vi "Main.vi"(8 "error in (no error)":errorcluster, 11 "ModuleAdmin":refnum<class "ModuleAdmin.lvclass">) -> ()   [LabVIEW 2014, in "WfrmModule.lvlib"]
uses:
  WfrmModule.lvlib
  <userlib>/NIST/ModuleAdminLib/ModuleAdmin/ModuleAdmin.lvclass
  PublicAPI/Arguments/Requests/clStopArgument.ctl
  PublicAPI/Arguments/Requests/clLoadPlugin.ctl
  WfrmPlugins/EventPluginBaseClass/BaseWfrmPlugin.lvclass
  <userlib>/NIST/ModuleAdminLib/ModuleAdmin/ModuleAdmin.lvclass/ModuleAdmin.ctl
  WfrmPlugins/EventPluginBaseClass/TypeDefs/WfrmConfig.ctl
  PublicAPI/Arguments/Requests/clTimeParams.ctl
  WfrmPlugins/EventPluginBaseClass/BaseWfrmPlugin.lvclass/BaseWfrmPlugin.ctl
  PublicAPI/Arguments/Requests/dblEvtParams.ctl
  WfrmPlugins/EventPluginBaseClass/TypeDefs/clWfrmParams.ctl
  <vilib>/Utility/error.llb/DialogType.ctl
  <userlib>/NIST/ModuleAdminLib/ModuleAdmin/Accessors/Read ShowPanel_.vi
  WfrmPlugins/EventPluginBaseClass/Accessors/Write StartTime.vi
  WfrmPlugins/EventPluginBaseClass/Accessors/Write EndTime.vi
  WfrmPlugins/EventPluginBaseClass/Accessors/Write SettlingTime.vi
  WfrmPlugins/EventPluginBaseClass/Accessors/Read StartTime.vi
  WfrmPlugins/EventPluginBaseClass/Accessors/Read EndTime.vi
  WfrmPlugins/EventPluginBaseClass/Accessors/Read SettlingTime.vi
  WfrmPlugins/EventPluginBaseClass/Accessors/Write clWfrmParams.vi
  WfrmPlugins/EventPluginBaseClass/Accessors/Read clWfrmParams.vi
  <userlib>/NIST/ModuleAdminLib/ModuleAdmin/Accessors/Write ShowPanel_.vi
  <userlib>/NIST/ModuleAdminLib/ModuleAdmin/Accessors/Read CloneRegRef.vi
  <vilib>/Utility/error.llb/Error Cluster From Error Code.vi
  <vilib>/Analysis/1siggen.llb/Ramp Pattern by Delta.vi
  <vilib>/ErrorRing/Error Ring.xnode
  <userlib>/NIST/ModuleAdminLib/CloneRegistration/CloneRegistration.lvclass
  <vilib>/Analysis/NI_AALBase.lvlib
  <userlib>/NIST/ModuleAdminLib/ModuleAdmin.lvlib
  <userlib>/NIST/BaseClasses/Object_class/BaseObject.lvclass
panel:
  out "error out":errorcluster
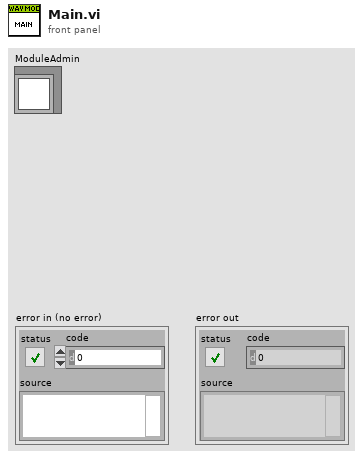
[diagram p1: front panel]
types:
  T1 = typedef "WfrmModule.lvlib/clRequestEvents.ctl" = cluster{"StopRequest":refnum<user-event>, "LoadPluginRequest":refnum<user-event>, "WriteEvtConfig":refnum<user-event>, "ReadEvtConfig":refnum<user-event>, "WriteTimeArray":refnum<user-event>, "ReadTimeArray":refnum<user-event>, "WriteEvtParams":refnum<user-event>, "ReadEvtParams":refnum<user-event>, "GetEvtReportArray":refnum<user-event>, "ReadPathToPlugin":refnum<user-event>, "GetEvtSignal":refnum<user-event>, "SendArbWfrm":refnum<user-event>, "ShowPanel":refnum<user-event>, "ReadWfrmParams":refnum<user-event>, "WriteWfrmParams":refnum<user-event>, "WriteStartEndTime":refnum<user-event>, "ConfigDlg":refnum<user-event>, "ReadStartEndSettlingTime":refnum<user-event>}
  T2 = typedef "WfrmModule.lvlib/clBroadcastEvents.ctl" = cluster{"DidInit":refnum<user-event>, "StatusUpdate":refnum<user-event>, "ErrorReport":refnum<user-event>, "DidStop":refnum<user-event>, "ReadEvtConfig":refnum<user-event>, "ReadTimeArray":refnum<user-event>, "ReadEvtParams":refnum<user-event>, "GetEvtReportArray":refnum<user-event>, "ReadPathToPlugin":refnum<user-event>, "GetEvtSignal":refnum<user-event>, "SendArbWfrm":refnum<user-event>, "WfrmParams":refnum<user-event>, "StartEndSettling":refnum<user-event>}
  T3 = typedef "WfrmModule.lvlib/clStopArgument.ctl" = cluster{"Exit via Stop Module Req?":bool, "Wait for Module to stop?":bool, "ModuleAdmin":refnum<class "ModuleAdmin.lvclass">}
  T4 = typedef "WfrmModule.lvlib/clLoadPlugin.ctl" = cluster{"PathToPlugin":path}
  T5 = enum32{"Invalid", "Standard", "Closed", "Hidden", "Minimized", "Maximized"}
  T6 = typedef "WfrmPlugins.lvlib/BaseWfrmPlugin.lvclass/WfrmConfig.ctl" = cluster{"T0(UTC)":dbl, "F0":dbl, "Fs":i32, "FSamp":u32}
  T7 = typedef "WfrmModule.lvlib/clTimeParams.ctl" = cluster{"dblTimeArray":dbl[], "StartTime":dbl, "EndTime":dbl, "SettlingTime":dbl}
  T8 = typedef "WfrmModule.lvlib/dblEvtParams.ctl" = dbl[][]
  T9 = typedef "WfrmPlugins.lvlib/BaseWfrmPlugin.lvclass/clWfrmParams.ctl" = cluster{"RowHdrs":string[], "ColHdrs":string[], "DefaultParams":string[][]}
  T10 = typedef "EventPlugins.lvlib/EventPluginBaseClass.lvclass/clEvtReportArray.ctl" = T11[]
  T11 = typedef "EventPlugins.lvlib/EventPluginBaseClass.lvclass/clEvtReport.ctl" = cluster{"Timestamp":dbl, "Synx":cdb[], "Freq":dbl, "ROCOF":dbl}
  T12 = typedef "EventModule.lvlib/dblEvtSignalArray.ctl" = dbl[][]
  T13 = typedef "DialogType.ctl" = u16
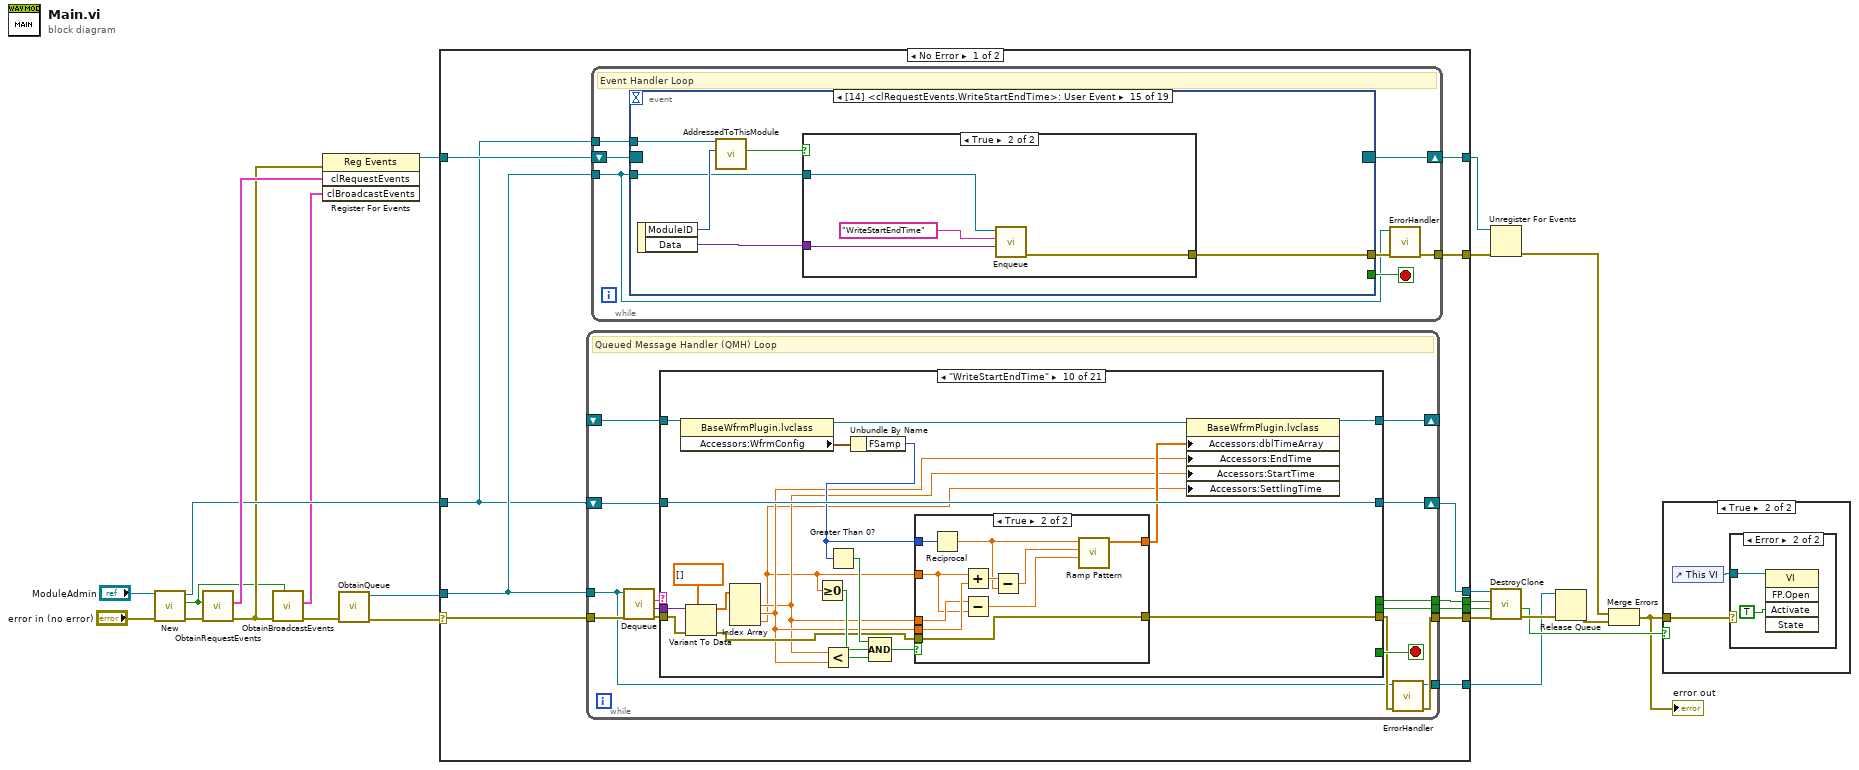
[diagram p0: block diagram]
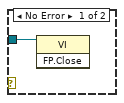
[diagram p3: hidden frame]
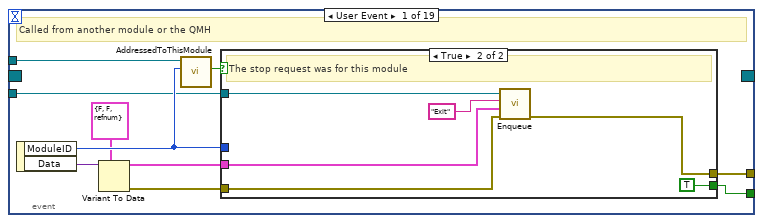
[diagram p4: hidden frame]
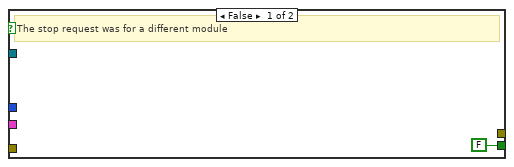
[diagram p5: hidden frame]
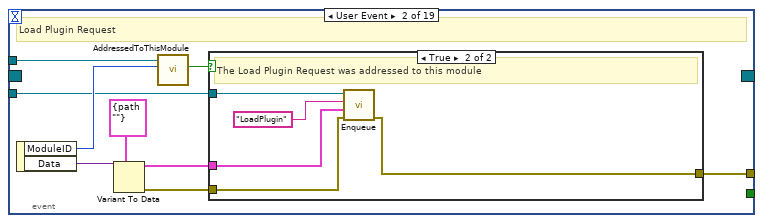
[diagram p6: hidden frame]
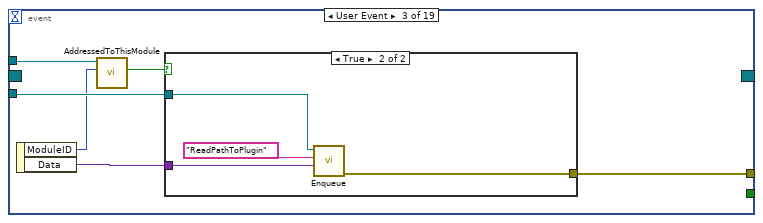
[diagram p8: hidden frame]
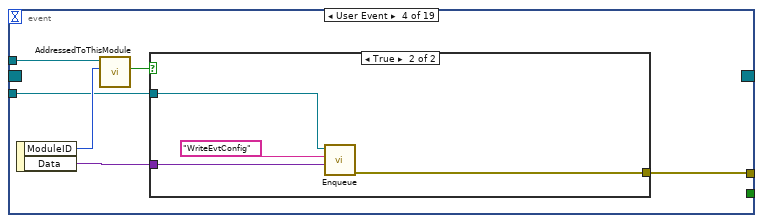
[diagram p10: hidden frame]
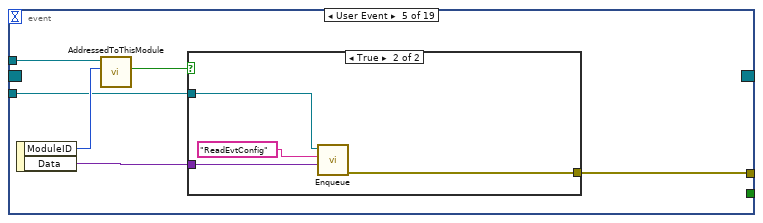
[diagram p12: hidden frame]
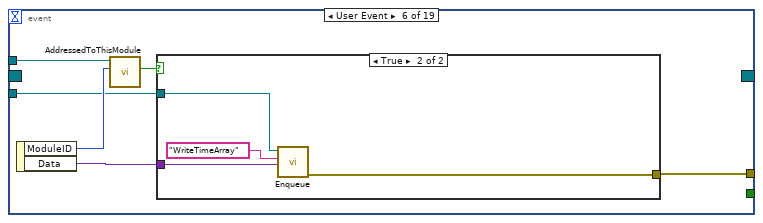
[diagram p14: hidden frame]
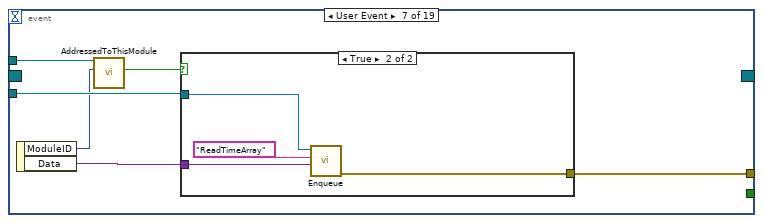
[diagram p16: hidden frame]
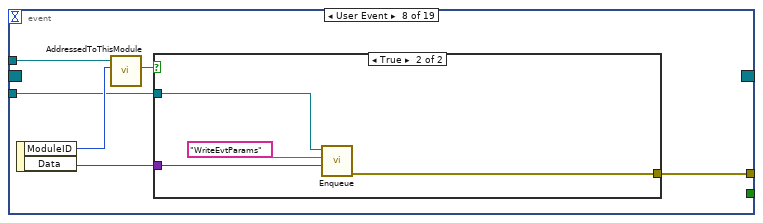
[diagram p18: hidden frame]
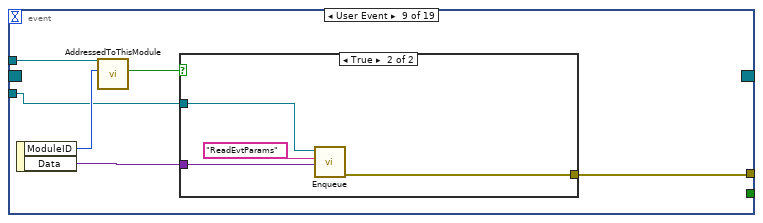
[diagram p20: hidden frame]
diagram:
  n1 = call <userlib>:"New.vi"("error in (no error)"="error in (no error)", "ModuleAdmin"="ModuleAdmin") -> ("error out"=w22:errorcluster, "First?"=w1:bool, "ModuleAdmin"=w18:refnum<class "ModuleAdmin.lvclass">)  [unwired: 7 in]
  n2 = call "ObtainRequestEvents.vi"("error in (no error)"=w22, "CreateNew (f)"=w1) -> ("error out"=w16:errorcluster, "clRequestEvents"=w21:T1)  [unwired: 8 in]
  n3 = call "ObtainBroadcastEvents.vi"("Init? (f)"=w1, "error in (no error)"=w16) -> ("error out"=w17:errorcluster, "clBroadcastEvents"=w15:T2)  [unwired: 8 in]
  n4 = register-events(error in=w16, w21, w15) -> (reference out=w14:refnum<event-registration>)  [unwired: 1 in, 1 out]
  n5 = call "ObtainQueue.vi"("error in (no error)"=w17) -> ("error out"=w20:errorcluster, "MessageQueue"=w19:refnum<queue>)  [unwired: 9 in]
  n6 = case shown="No Error" w20 {
    selector: w20 -> [w35 w635]
    tunnel: w19 -> [w33 w630]
    tunnel: w18 -> [w26 w632]
    tunnel: [w34 w633] -> w13
    tunnel: w14 -> [w32 w627]
    tunnel: [w31 w631] -> w11
    tunnel: [w30 _] -> w10
    tunnel: [w29 _] -> w9
    tunnel: [w28 _] -> w5
    tunnel: [w27 w630] -> w6
    tunnel: [w25 w627] -> w4
    frame No Error {
      n7 = while {
        tunnel: w33 -> [w252]
        tunnel: w35 -> [w260]
        tunnel: [w254] -> w34
        tunnel: [w256] -> w30
        tunnel: [w255] -> w29
        tunnel: [w251] -> w27
        shift-right: [w250] -> _
        shift-left: _ -> [w249]
        shift-right: [w248] -> w31
        shift-left: w26 -> [w247]
        stop <- w261 stop-if-true
        # "Queued Message Handler (QMH) Loop"
        n8 = call "Dequeue.vi"("error in (no error)"=w260, "MessageQueue"=w252) -> ("error out"=w259:errorcluster, "Message Data"=w257:variant, "Message"=w258:string)  [unwired: 6 in, 1 out]
        n9 = case shown="\"WriteStartEndTime\"" w258 {
          selector: w258 -> [w266 _ _ _ _ _ _ _ _ _ _ _ _ _ _ _ _ _ _ _ _]
          tunnel: [_ _ _ _ _ _ _ _ _ _ _ _ _ _ _ _ _ _ _ TRUE _] -> w261
          tunnel: w247 -> [w269 w298 w310 w359 w363 w375 w388 w399 w442 w467 w496 w508 w524 w535 w545 w562 w575 w588 w593 w601 w621]
          tunnel: [w265 w287 w311 w356 w365 w377 w386 w398 w441 w453 w498 w507 w523 w534 w544 w552 w565 w581 w591 w608 w612] -> w253
          tunnel: w259 -> [_ _ w321 w358 w367 w379 w383 w400 w443 w462 w499 w509 w525 w536 w546 w561 w574 w587 w599 w607 w620]
          tunnel: w257 -> [_ _ w325 _ _ w380 _ w401 _ w463 _ w510 w526 _ _ _ _ _ w600 w606 w619]
          tunnel: [_ _ _ _ _ _ _ _ _ _ _ _ _ _ _ _ _ _ _ w604 _] -> w256
          tunnel: [_ _ _ _ _ _ _ _ _ _ _ _ _ _ _ _ _ _ _ w603 _] -> w255
          tunnel: [w263 refnum<class "BaseWfrmPlugin.lvclass"> refnum ("EventPlugins.lvlib:EventPluginBaseClass.lvclass") w315 w357 w364 w376 w387 w397 w444 w465 w493 w505 w521 w533 w543 w558 w571 w584 w589 w602 w611] -> w250
          tunnel: w249 -> [w263 _ w316 w360 w366 w370 w389 w396 w445 w466 w503 w506 w522 w537 w547 w560 w573 w586 w589 w602 w611]
          tunnel: [w262 w282 w309 w354 w363 w368 w381 w392 w439 w467 w495 w504 w520 w532 w542 w550 w563 w576 w590 w601 w610] -> w248
          frame Default {
            n10 = property class="ModuleAdmin.lvclass"(reference=w269) -> (reference out=w262:refnum<class "ModuleAdmin.lvclass">, "Accessors:Module ID"=w268:i32, "Accessors:ModuleName"=w264:string)  [unwired: 1 in, 1 out]
            n11 = call <userlib>:"ModuleName.vi"("Name"=w264, "ModuleID"=w268) -> ("ModuleName"=w267:string)  [unwired: 9 in]
            n12 = xnode "Error Ring"("parameter 0"=w266, "parameter 1"=w267) -> ("error out"=w265:errorcluster)
          }
          frame "Initialize" {
            n13 = property class="ModuleAdmin.lvclass"(reference=w298) -> (reference out=w283:refnum<class "ModuleAdmin.lvclass">, error out=w295:errorcluster, "Accessors:Module ID"=w286:i32, "Accessors:ShowPanel_"=w280:bool, "Accessors:External Launch"=w279:bool, "Accessors:ModuleName"=w281:string)  [unwired: 1 in]
            n14 = Compound Arithmetic op=OR(w280, invert w279) -> (w278:bool)
            n15 = Select(t=T5."Standard" ("Front Panel Window:State"), s=w278, f=T5."Hidden" ("Front Panel Window:State")) -> (s? t:f=w291:T5)
            n16 = invoke class="VI" method="FP.Open"(error in=w295, "State"=w291) -> (error out=w294:errorcluster)  [unwired: 3 in, 4 out]
            n17 = call <userlib>:"ModuleName.vi"("Name"=w281, "ModuleID"=w286) -> ("ModuleName"=w290:string)  [unwired: 9 in]
            n18 = property class="VI"(error in=w294, "Front Panel.Title"=w290) -> (reference out=w297:refnum<vi>, error out=w296:errorcluster)  [unwired: 1 in]
            n19 = invoke class="VI" method="FP.Center"(reference=w297, error in=w296) -> (error out=w285:errorcluster)  [unwired: 1 in, 2 out]
            n20 = case shown="True" w279 {
              tunnel: [w299 w305] -> w288
              tunnel: [w300 w302] -> w282
              tunnel: w285 -> [w299 w304]
              tunnel: w283 -> [w300 w301]
              frame False {
              }
              frame True {
                n21 = call <userlib>:"WaitOnModuleSync.vi"("error in (no error)"=w304, "ModuleAdmin"=w301) -> ("error out"=w306:errorcluster, "ModuleAdmin"=w303:refnum<class "ModuleAdmin.lvclass">)  [unwired: 8 in]
                n22 = call <userlib>:"WaitOnEventSync.vi"("error in (no error)"=w306, "ModuleAdmin"=w303) -> ("error out"=w305:errorcluster, "ModuleAdmin"=w302:refnum<class "ModuleAdmin.lvclass">)  [unwired: 8 in]
              }
            }
            n23 = call "DidInit.vi"("Init?"=TRUE, "error in (no error)"=w288, "ModuleAdmin"=w282) -> ("error out"=w287:errorcluster)  [unwired: 8 in]
          }
          frame "LoadPlugin" {
            n24 = Variant To Data(error in=w321, type=T4 {"PathToPlugin"=path ""} ("clLoadPlugin"), Variant=w325) -> (data=w323:T4, error out=w322:errorcluster)
            n25 = Unbundle By Name(w323) -> ("PathToPlugin"=w308:path)
            n26 = call <userlib>:"GetPathToClass.vi"("error in (no error)"=w322, "configuration file path"=w308) -> ("error IO"=w320:errorcluster, "PathToClass"=w312:path)  [unwired: 8 in]
            n27 = Current VI's Path() -> (path=w313:path)
            n28 = Build Path(base path=w313, name or relative path=w312) -> (appended path=w314:path)
            n29 = call <vilib>:"Check if File or Folder Exists.vi"("error in (no error)"=w320, "path"=w314) -> ("error out"=w318:errorcluster, "file or folder exists?"=w319:bool, "dup path"=w317:path)  [unwired: 7 in]
            n30 = case shown="True" w319 {
              tunnel: w317 -> [w335 w342]
              tunnel: w318 -> [w339 w345]
              tunnel: [w334 w346] -> w311
              tunnel: w316 -> [_ w340]
              tunnel: w310 -> [w331 w341]
              tunnel: [w330 w341] -> w309
              tunnel: w308 -> [w327 _]
              tunnel: [w326 w340] -> w307
              frame True {
                n31 = call-dynamic "LoadClassFromFile.vi"("error in (no error)"=w339, "class path"=w335, "reference in"=refnum<class "BaseWfrmPlugin.lvclass"> refnum ("EventPlugins.lvlib:EventPluginBaseClass.lvclass")) -> ("error out"=w329:errorcluster, "reference out"=w328:refnum<class "BaseWfrmPlugin.lvclass">)  [unwired: 7 in]
                n32 = property class="ModuleAdmin.lvclass"(reference=w331) -> (reference out=w330:refnum<class "ModuleAdmin.lvclass">, "Accessors:Module ID"=w332:i32)  [unwired: 1 in, 1 out]
                n33 = call-dynamic "GetDefaultParams.vi"("error in (no error)"=w329, "ConfigFilePath"=w327, "BaseWfrmPlugin in"=w328) -> ("BaseWfrmPlugin out"=w326:refnum<class "BaseWfrmPlugin.lvclass">)  [unwired: 7 in, 1 out]
                n34 = Path To String(path=w335) -> (string=w337:string)
                n35 = Format Into String(format string="Plugin %s loaded", w337) -> (resulting string=w333:string)  [unwired: 2 in, 1 out]
                n36 = call "StatusUpdate.vi"("Status"=w333, "ModuleID"=w332) -> ("error out"=w334:errorcluster)  [unwired: 9 in]
              }
              frame False {
                n37 = Path To String(path=w342) -> (string=w343:string)
                n38 = xnode "Error Ring"("parameter 0"=w343) -> ("error out"=w344:errorcluster)
                n39 = Merge Errors(w344, w345) -> (w346:errorcluster)
              }
            }
            n40 = property class="BaseWfrmPlugin.lvclass"(reference=w307, "Accessors:EvtPluginINIFilePath"=w308) -> (reference out=w315:refnum<class "BaseWfrmPlugin.lvclass">)  [unwired: 1 in, 1 out]
          }
          frame "ReadPathToPlugin" {
            n41 = property class="BaseWfrmPlugin.lvclass"(reference=w360, error in=w358) -> (reference out=w357:refnum<class "BaseWfrmPlugin.lvclass">, error out=w361:errorcluster, "Accessors:EvtPluginINIFilePath"=w355:path)
            n42 = property class="ModuleAdmin.lvclass"(reference=w359) -> (reference out=w354:refnum<class "ModuleAdmin.lvclass">, "Accessors:Module ID"=w362:i32)  [unwired: 1 in, 1 out]
            n43 = call "ReadPathToPlugin.vi"("error in (no error)"=w361, "EvtPluginINIFilePath"=w355, "ModuleID"=w362) -> ("error out"=w356:errorcluster)  [unwired: 8 in]
          }
          frame "ConfigDlg" {
            n44 = call "ConfigureDlg.vi"("error in (no error)"=w367, "BaseWfrmPlugin in"=w366) -> ("error out"=w365:errorcluster, "BaseWfrmPlugin out"=w364:refnum<class "BaseWfrmPlugin.lvclass">)  [unwired: 8 in]
          }
          frame "WriteEvtConfig" {
            n45 = Variant To Data(error in=w379, type=T6 {"T0(UTC)"=0.0, "F0"=0.0, "Fs"=0, "FSamp"=0} ("clEvtConfig"), Variant=w380) -> (data=w371:T6, error out=w369:errorcluster)
            n46 = property class="BaseWfrmPlugin.lvclass"(reference=w370, error in=w369, "Accessors:WfrmConfig"=w371) -> (reference out=w376:refnum<class "BaseWfrmPlugin.lvclass">, error out=w372:errorcluster)
            n47 = property class="ModuleAdmin.lvclass"(reference=w375) -> (reference out=w368:refnum<class "ModuleAdmin.lvclass">, "Accessors:Module ID"=w374:i32)  [unwired: 1 in, 1 out]
            n48 = call "StatusUpdate.vi"("error in (no error)"=w372, "Status"="Event Configuration Received", "ModuleID"=w374) -> ("error out"=w377:errorcluster)  [unwired: 8 in]
          }
          frame "ReadEvtConfig" {
            n49 = property class="BaseWfrmPlugin.lvclass"(reference=w389, error in=w383) -> (reference out=w387:refnum<class "BaseWfrmPlugin.lvclass">, error out=w384:errorcluster, "Accessors:WfrmConfig"=w382:T6)
            n50 = property class="ModuleAdmin.lvclass"(reference=w388) -> (reference out=w381:refnum<class "ModuleAdmin.lvclass">, "Accessors:Module ID"=w385:i32)  [unwired: 1 in, 1 out]
            n51 = call "ReadEvtConfig.vi"("error in (no error)"=w384, "WfrmConfigReport"=w382, "ModuleID"=w385) -> ("error out"=w386:errorcluster)  [unwired: 8 in]
          }
          frame "WriteTimeArray" {
            n52 = Variant To Data(error in=w400, type=T7 {"dblTimeArray"=[], "StartTime"=0.0, "EndTime"=0.0, "SettlingTime"=7.0} ("clTimeParams"), Variant=w401) -> (data=w393:T7, error out=w395:errorcluster)
            n53 = Unbundle By Name(w393) -> ("dblTimeArray"=w390:dbl[])
            n54 = Array Size(array=w390) -> (size(s)=w394:i32)
            n55 = case shown="Default" w394 {
              tunnel: w399 -> [w409 w437]
              tunnel: [w412 w436] -> w398
              tunnel: [w419 w435] -> w397
              tunnel: w396 -> [w418 w432]
              tunnel: w395 -> [_ w431]
              tunnel: w393 -> [_ w430]
              tunnel: [w402 w429] -> w392
              frame 0, 1 {
                w415 = 0.0  # StartTime
                w416 = 1.0  # EndTime
                # "If the time array does not contain a valid time interval, set default time array and throw 5102 error."
                n56 = property class="BaseWfrmPlugin.lvclass"(reference=w418) -> (reference out=w417:refnum<class "BaseWfrmPlugin.lvclass">, error out=w414:errorcluster, "Accessors:WfrmConfig"=w405:T6)  [unwired: 1 in]
                n57 = property class="ModuleAdmin.lvclass"(reference=w409) -> (reference out=w402:refnum<class "ModuleAdmin.lvclass">, "Accessors:Module ID"=w408:i32)  [unwired: 1 in, 1 out]
                n58 = xnode "Error Ring"() -> ("error out"=w411:errorcluster)
                n59 = Unbundle By Name(w405) -> ("Fs"=w404:i32)
                n60 = Reciprocal(x=w404) -> (1/x=w406:dbl)
                n61 = call-poly <vilib>:"Ramp Pattern.vi"("start"=w415, "end"=w416, "delta"=w406) -> ("Ramp Pattern"=w403:dbl[])  [unwired: 6 in, 2 out]
                n62 = property class="BaseWfrmPlugin.lvclass"(reference=w417, error in=w414, "Accessors:dblTimeArray"=w403) -> (reference out=w419:refnum<class "BaseWfrmPlugin.lvclass">, error out=w410:errorcluster)
                n63 = call "StatusUpdate.vi"("error in (no error)"=w410, "Status"="Time Array invalid, setting 0 to 1 sec interval", "ModuleID"=w408) -> ("error out"=w413:errorcluster)  [unwired: 8 in]
                n64 = Merge Errors(w413, w411) -> (w412:errorcluster)
              }
              frame Default {
                n65 = Unbundle By Name(w430) -> ("dblTimeArray"=w428:dbl[], "StartTime"=w427:dbl, "EndTime"=w426:dbl, "SettlingTime"=w425:dbl)
                n66 = property class="BaseWfrmPlugin.lvclass"(reference=w432, error in=w431, "Accessors:dblTimeArray"=w428, "Accessors:StartTime"=w427, "Accessors:EndTime"=w426, "Accessors:SettlingTime"=w425) -> (reference out=w435:refnum<class "BaseWfrmPlugin.lvclass">, error out=w434:errorcluster)
                n67 = property class="ModuleAdmin.lvclass"(reference=w437) -> (reference out=w429:refnum<class "ModuleAdmin.lvclass">, "Accessors:Module ID"=w433:i32)  [unwired: 1 in, 1 out]
                n68 = call "StatusUpdate.vi"("error in (no error)"=w434, "Status"="Time Array Received", "ModuleID"=w433) -> ("error out"=w436:errorcluster)  [unwired: 8 in]
              }
            }
          }
          frame "ReadTimeArray" {
            n69 = property class="BaseWfrmPlugin.lvclass"(reference=w445, error in=w443) -> (reference out=w444:refnum<class "BaseWfrmPlugin.lvclass">, error out=w446:errorcluster, "Accessors:dblTimeArray"=w440:dbl[])
            n70 = property class="ModuleAdmin.lvclass"(reference=w442) -> (reference out=w439:refnum<class "ModuleAdmin.lvclass">, "Accessors:Module ID"=w447:i32)  [unwired: 1 in, 1 out]
            n71 = call "ReadTimeArray.vi"("error in (no error)"=w446, "dblTime Array"=w440, "ModuleID"=w447) -> ("error out"=w441:errorcluster)  [unwired: 8 in]
          }
          frame "WriteStartEndTime" {
            n72 = property class="BaseWfrmPlugin.lvclass"(reference=w466) -> (reference out=w464:refnum<class "BaseWfrmPlugin.lvclass">, "Accessors:WfrmConfig"=w459:T6)  [unwired: 1 in, 1 out]
            n73 = Variant To Data(error in=w462, type=dbl[] [], Variant=w463) -> (data=w460:dbl[], error out=w451:errorcluster)
            n74 = Index Array(array=w460) -> (element #1=w449:dbl, element #2=w450:dbl, element #3=w448:dbl)  [unwired: 3 in]
            n75 = Greater Or Equal To 0?(x=w448) -> (x >= 0?=w457:bool)
            n76 = Less?(x=w449, y=w450) -> (x < y?=w458:bool)
            n77 = Unbundle By Name(w459) -> ("FSamp"=w454:u32)
            n78 = Greater Than 0?(x=w454) -> (x > 0?=w456:bool)
            n79 = Compound Arithmetic op=AND(w456, w457, w458) -> (w455:bool)
            n80 = case shown="True" w455 {
              tunnel: w454 -> [w470 w492]
              tunnel: w448 -> [w469 w487]
              tunnel: w449 -> [w472 w488]
              tunnel: w450 -> [w471 w491]
              tunnel: [w468 w483] -> w453
              tunnel: [_ w484] -> w452
              tunnel: w451 -> [_ w483]
              frame False {
                n81 = xnode "Error Ring"("parameter 0"=w472, "parameter 1"=w471, "parameter 2"=w470, "parameter 3"=w469) -> ("error out"=w468:errorcluster)
              }
              frame True {
                n82 = Reciprocal(x=w492) -> (1/x=w489:dbl)
                n83 = Add(x=w487, y=w491) -> (x+y=w490:dbl)
                n84 = Subtract(x=w488, y=w487) -> (x-y=w485:dbl)
                n85 = Subtract(x=w490, y=w489) -> (x-y=w486:dbl)
                n86 = call-poly <vilib>:"Ramp Pattern.vi"("start"=w485, "end"=w486, "delta"=w489) -> ("Ramp Pattern"=w484:dbl[])  [unwired: 6 in, 2 out]
              }
            }
            n87 = property class="BaseWfrmPlugin.lvclass"(reference=w464, "Accessors:dblTimeArray"=w452, "Accessors:EndTime"=w450, "Accessors:StartTime"=w449, "Accessors:SettlingTime"=w448) -> (reference out=w465:refnum<class "BaseWfrmPlugin.lvclass">)  [unwired: 1 in, 1 out]
          }
          frame "ReadStartEndTime" {
            n88 = property class="BaseWfrmPlugin.lvclass"(reference=w503) -> (reference out=w493:refnum<class "BaseWfrmPlugin.lvclass">, "Accessors:StartTime"=w500:dbl, "Accessors:EndTime"=w501:dbl, "Accessors:SettlingTime"=w502:dbl)  [unwired: 1 in, 1 out]
            n89 = property class="ModuleAdmin.lvclass"(reference=w496) -> (reference out=w495:refnum<class "ModuleAdmin.lvclass">, "Accessors:Module ID"=w494:i32)  [unwired: 1 in, 1 out]
            n90 = Build Array(w500, w501, w502) -> (w497:dbl[])
            n91 = call "ReadStartEndSettling.vi"("error in (no error)"=w499, "StartEndSettling"=w497, "ModuleID"=w494) -> ("error out"=w498:errorcluster)  [unwired: 8 in]
          }
          frame "WriteEvtParams" {
            w511 = T8 []  # SignalParams
            # "Can't change \"SignalParams\" to icon."
            n92 = Variant To Data(error in=w509, type=w511, Variant=w510) -> (data=w512:T8, error out=w516:errorcluster)
            n93 = property class="BaseWfrmPlugin.lvclass"(reference=w506, error in=w516, "Accessors:dblEvtParams"=w512) -> (reference out=w505:refnum<class "BaseWfrmPlugin.lvclass">, error out=w513:errorcluster)
            n94 = property class="ModuleAdmin.lvclass"(reference=w508) -> (reference out=w504:refnum<class "ModuleAdmin.lvclass">, "Accessors:Module ID"=w515:i32)  [unwired: 1 in, 1 out]
            n95 = call "StatusUpdate.vi"("error in (no error)"=w513, "Status"="Event Parameters Received", "ModuleID"=w515) -> ("error out"=w507:errorcluster)  [unwired: 8 in]
          }
          frame "WriteWfrmParams" {
            w527 = T9 {"RowHdrs"=[], "ColHdrs"=[], "DefaultParams"=[]}  # SignalParams
            n96 = Variant To Data(error in=w525, type=w527, Variant=w526) -> (data=w518:T9, error out=w531:errorcluster)
            n97 = Unbundle By Name(w518) -> ("DefaultParams"=w517:string[][])
            n98 = call "Tbl2Array.vi"("strTable"=w517) -> ("dblArray"=w519:dbl[][])  [unwired: 10 in]
            n99 = property class="BaseWfrmPlugin.lvclass"(reference=w522, error in=w531, "Accessors:clWfrmParams"=w518, "Accessors:dblEvtParams"=w519) -> (reference out=w521:refnum<class "BaseWfrmPlugin.lvclass">, error out=w528:errorcluster)
            n100 = property class="ModuleAdmin.lvclass"(reference=w524) -> (reference out=w520:refnum<class "ModuleAdmin.lvclass">, "Accessors:Module ID"=w530:i32)  [unwired: 1 in, 1 out]
            n101 = call "StatusUpdate.vi"("error in (no error)"=w528, "Status"="Waveform Parameters Received", "ModuleID"=w530) -> ("error out"=w523:errorcluster)  [unwired: 8 in]
          }
          frame "ReadEvtParams" {
            n102 = property class="BaseWfrmPlugin.lvclass"(reference=w537, error in=w536) -> (reference out=w533:refnum<class "BaseWfrmPlugin.lvclass">, error out=w539:errorcluster, "Accessors:dblEvtParams"=w538:dbl[][])
            n103 = property class="ModuleAdmin.lvclass"(reference=w535) -> (reference out=w532:refnum<class "ModuleAdmin.lvclass">, "Accessors:Module ID"=w540:i32)  [unwired: 1 in, 1 out]
            n104 = call "ReadEvtParams.vi"("error in (no error)"=w539, "SignalParams"=w538, "ModuleID"=w540) -> ("error out"=w534:errorcluster)  [unwired: 8 in]
          }
          frame "ReadWfrmParams" {
            n105 = property class="BaseWfrmPlugin.lvclass"(reference=w547, error in=w546) -> (reference out=w543:refnum<class "BaseWfrmPlugin.lvclass">, error out=w548:errorcluster, "Accessors:clWfrmParams"=w541:T9)
            n106 = property class="ModuleAdmin.lvclass"(reference=w545) -> (reference out=w542:refnum<class "ModuleAdmin.lvclass">, "Accessors:Module ID"=w549:i32)  [unwired: 1 in, 1 out]
            n107 = call "WfrmParams.vi"("error in (no error)"=w548, "WfrmParams"=w541, "ModuleID"=w549) -> ("error out"=w544:errorcluster)  [unwired: 8 in]
          }
          frame "GetReportArray" {
            n108 = call-dynamic "GetEvtReports.vi"("error in (no error)"=w561, "EventPluginBaseClass in"=w560) -> ("error out"=w557:errorcluster, "EventPluginBaseClass out"=w559:refnum<class "BaseWfrmPlugin.lvclass">)  [unwired: 8 in]
            n109 = property class="ModuleAdmin.lvclass"(reference=w562) -> (reference out=w550:refnum<class "ModuleAdmin.lvclass">, "Accessors:Module ID"=w551:i32)  [unwired: 1 in, 1 out]
            n110 = property class="BaseWfrmPlugin.lvclass"(reference=w559, error in=w557) -> (reference out=w558:refnum<class "BaseWfrmPlugin.lvclass">, error out=w556:errorcluster, "Accessors:clEvtReportArray"=w555:T10)
            n111 = call "GetEvtReports.vi"("error in (no error)"=w556, "clReportArray"=w555, "ModuleID"=w551) -> ("error out"=w553:errorcluster)  [unwired: 8 in]
            n112 = call "StatusUpdate.vi"("error in (no error)"=w553, "Status"="Event Reports Transmitted", "ModuleID"=w551) -> ("error out"=w552:errorcluster)  [unwired: 8 in]
          }
          frame "GetEvtSignal" {
            n113 = call-dynamic "GetEvtSignal.vi"("error in (no error)"=w574, "EventPluginBaseClass in"=w573) -> ("error out"=w570:errorcluster, "EventPluginBaseClass out"=w572:refnum<class "BaseWfrmPlugin.lvclass">)  [unwired: 8 in]
            n114 = property class="ModuleAdmin.lvclass"(reference=w575) -> (reference out=w563:refnum<class "ModuleAdmin.lvclass">, "Accessors:Module ID"=w564:i32)  [unwired: 1 in, 1 out]
            n115 = property class="BaseWfrmPlugin.lvclass"(reference=w572, error in=w570) -> (reference out=w571:refnum<class "BaseWfrmPlugin.lvclass">, error out=w569:errorcluster, "Accessors:dblEventSignalArray"=w568:T12)
            n116 = call "GetEvtSignal.vi"("error in (no error)"=w569, "clReportArray"=w568, "ModuleID"=w564) -> ("error out"=w566:errorcluster)  [unwired: 8 in]
            n117 = call "StatusUpdate.vi"("error in (no error)"=w566, "Status"="Event Signal Transmitted", "ModuleID"=w564) -> ("error out"=w565:errorcluster)  [unwired: 8 in]
          }
          frame "SendArbWfrm" {
            n118 = call-dynamic "GetEvtSignal.vi"("error in (no error)"=w587, "EventPluginBaseClass in"=w586) -> ("error out"=w583:errorcluster, "EventPluginBaseClass out"=w585:refnum<class "BaseWfrmPlugin.lvclass">)  [unwired: 8 in]
            n119 = property class="ModuleAdmin.lvclass"(reference=w588) -> (reference out=w576:refnum<class "ModuleAdmin.lvclass">, "Accessors:Module ID"=w580:i32)  [unwired: 1 in, 1 out]
            n120 = property class="BaseWfrmPlugin.lvclass"(reference=w585, error in=w583) -> (reference out=w584:refnum<class "BaseWfrmPlugin.lvclass">, error out=w578:errorcluster, "Accessors:dblEventSignalArray"=w579:T12)
            n121 = call "SendEvtSignal.vi"("error in (no error)"=w578, "clReportArray"=w579, "ModuleID"=w580) -> ("error out"=w577:errorcluster)  [unwired: 8 in]
            n122 = call "StatusUpdate.vi"("error in (no error)"=w577, "Status"="Event Signal Transmitted", "ModuleID"=w580) -> ("error out"=w581:errorcluster)  [unwired: 8 in]
          }
          frame "ShowPanel" {
            n123 = Variant To Data(error in=w599, type=TRUE, Variant=w600) -> (data=w592:bool, error out=w594:errorcluster)
            n124 = Select(t=T5."Standard" ("Front Panel Window:State"), s=w592, f=T5."Hidden" ("Front Panel Window:State")) -> (s? t:f=w595:T5)
            n125 = property class="VI"(error in=w594, "FP.State"=w595) -> (error out=w591:errorcluster)  [unwired: 1 in, 1 out]
            n126 = property class="ModuleAdmin.lvclass"(reference=w593, "Accessors:ShowPanel_"=w592) -> (reference out=w590:refnum<class "ModuleAdmin.lvclass">)  [unwired: 1 in, 1 out]
          }
          frame "Exit" {
            n127 = control-ref of="This VI"() -> (w605:refnum<vi>)
            n128 = call "HandleExit.vi"("error in (no error)"=w607, "VI Refnum"=w605, "StopArgument"=w606, "ModuleAdmin"=w601) -> ("error out"=w608:errorcluster, "Exit via Stop Module Req?"=w603:bool, "WaitForStop?"=w604:bool)  [unwired: 5 in]
          }
          frame "Error" {
            n129 = property class="ModuleAdmin.lvclass"(reference=w621) -> (reference out=w610:refnum<class "ModuleAdmin.lvclass">, "Accessors:External Launch"=w615:bool, "Accessors:Module ID"=w613:i32)  [unwired: 1 in, 1 out]
            n130 = Variant To Data(error in=w620, type=errorcluster {"status"=FALSE, "code"=0, "source"=""} ("error constant"), Variant=w619) -> (data=w614:errorcluster, error out=w617:errorcluster)
            n131 = call "ReportError.vi"("error in (no error)"=w617, "ErrorReported"=w614, "ModuleID"=w613) -> ("error out"=w616:errorcluster)  [unwired: 8 in]
            n132 = case shown="True" w615 {
              tunnel: w616 -> [w625 w626]
              tunnel: w614 -> [w624 _]
              tunnel: [w623 w626] -> w612
              tunnel: w610 -> [w622 _]
              frame False {
                # "Todo:  Add an event to ask the user\nIf the module should stop or continue"
                # "Stand alone: now, force an exit"
                n133 = call <vilib>:"Simple Error Handler.vi"("error in (no error)"=w624) -> ()  [unwired: 4 in, 5 out]
                n134 = call "StopRequest.vi"("error in (no error)"=w625, "ModuleAdmin"=w622) -> ("error out"=w623:errorcluster)  [unwired: 8 in, 1 out]
              }
              frame True {
                # "Externally launched modules only broadcast the error msg"
              }
            }
          }
        }
        n135 = call "ErrorHandler.vi"("error in (no error)"=w253, "MessageQueue"=w252) -> ("error out"=w254:errorcluster, "MessageQueue"=w251:refnum<queue>)  [unwired: 8 in]
      }
      n136 = while {
        tunnel: w33 -> [w36]
        shift-right: [w40] -> w25
        shift-left: w32 -> [w41]
        tunnel: w26 -> [w39]
        tunnel: [w37] -> w28
        stop <- w42 stop-if-true
        # "Event Handler Loop"
        n137 = event shown="[14] <clRequestEvents.WriteStartEndTime>: User Event" {
          selector: w41 -> [_ _ _ _ _ _ _ _ _ _ _ _ _ _ _ _ _ _ _]
          dyn-events: [_ _ _ _ _ _ _ _ _ _ _ _ _ _ _ _ _ _ _] -> w40
          timeout: _ -> [_ _ _ _ _ _ _ _ _ _ _ _ _ _ _ _ _ _ _]
          tunnel: w36 -> [w49 w63 w77 w85 w95 w104 w117 w125 w135 w145 w155 w166 w176 w186 w196 w206 w216 w226 w246]
          tunnel: [w48 _ _ _ _ _ _ _ _ _ _ _ _ _ _ _ _ _ TRUE] -> w42
          tunnel: w39 -> [w52 w60 w78 w88 w99 w107 w118 w126 w137 w147 w157 w168 w178 w188 w198 w208 w218 w229 w240]
          tunnel: [w47 w62 w74 w84 w94 w108 w114 w124 w134 w144 w154 w164 w174 w184 w194 w204 w214 w224 w244] -> w38
          event User Event {
            # "Called from another module or the QMH"
            n138 = event-data() -> ("ModuleID"=w50:i32, "Data"=w46:variant)  [unwired: 1 in]
            n139 = Variant To Data(type=T3 {"Exit via Stop Module Req?"=FALSE, "Wait for Module to stop?"=FALSE, "ModuleAdmin"=refnum} ("Stop Argument"), Variant=w46) -> (data=w44:T3, error out=w43:errorcluster)  [unwired: 1 in]
            n140 = call <userlib>:"AddressedToThisModule.vi"("ModuleID"=w50, "ModuleAdmin"=w52) -> ("AddressedToThisInstance?"=w51:bool)  [unwired: 8 in, 1 out]
            n141 = case shown="True" w51 {
              tunnel: w50 -> [_ _]
              tunnel: w49 -> [_ w59]
              tunnel: [FALSE TRUE] -> w48
              tunnel: [_ w57] -> w47
              tunnel: w44 -> [_ w55]
              tunnel: w43 -> [_ w54]
              frame False {
                # "The stop request was for a different module"
              }
              frame True {
                # "The stop request was for this module"
                n142 = call "Enqueue.vi"("error in (no error)"=w54, "Message Data"=w55, "Message"="Exit", "MessageQueue"=w59) -> ("error out"=w57:errorcluster)  [unwired: 6 in, 1 out]
              }
            }
          }
          event User Event {
            # "Load Plugin Request"
            n143 = event-data() -> ("ModuleID"=w64:i32, "Data"=w68:variant)  [unwired: 1 in]
            n144 = Variant To Data(type=T4 {"PathToPlugin"=path ""} ("clLoadPlugin"), Variant=w68) -> (data=w65:T4, error out=w61:errorcluster)  [unwired: 1 in]
            n145 = call <userlib>:"AddressedToThisModule.vi"("ModuleID"=w64, "ModuleAdmin"=w60) -> ("AddressedToThisInstance?"=w66:bool)  [unwired: 8 in, 1 out]
            n146 = case shown="True" w66 {
              tunnel: w65 -> [_ w73]
              tunnel: w63 -> [_ w72]
              tunnel: [_ w70] -> w62
              tunnel: w61 -> [_ w69]
              frame False {
                # "Not addressed to this module"
              }
              frame True {
                # "The Load Plugin Request was addressed to this module"
                n147 = call "Enqueue.vi"("error in (no error)"=w69, "Message Data"=w73, "Message"="LoadPlugin", "MessageQueue"=w72) -> ("error out"=w70:errorcluster)  [unwired: 6 in, 1 out]
              }
            }
          }
          event User Event {
            n148 = event-data() -> ("ModuleID"=w76:i32, "Data"=w75:variant)  [unwired: 1 in]
            n149 = call <userlib>:"AddressedToThisModule.vi"("ModuleID"=w76, "ModuleAdmin"=w78) -> ("AddressedToThisInstance?"=w79:bool)  [unwired: 8 in, 1 out]
            n150 = case shown="True" w79 {
              tunnel: w75 -> [_ w83]
              tunnel: w77 -> [_ w82]
              tunnel: [_ w80] -> w74
              frame False {
              }
              frame True {
                n151 = call "Enqueue.vi"("Message Data"=w83, "Message"="ReadPathToPlugin", "MessageQueue"=w82) -> ("error out"=w80:errorcluster)  [unwired: 7 in, 1 out]
              }
            }
          }
          event User Event {
            n152 = event-data() -> ("ModuleID"=w89:i32, "Data"=w86:variant)  [unwired: 1 in]
            n153 = call <userlib>:"AddressedToThisModule.vi"("ModuleID"=w89, "ModuleAdmin"=w88) -> ("AddressedToThisInstance?"=w87:bool)  [unwired: 8 in, 1 out]
            n154 = case shown="True" w87 {
              tunnel: w86 -> [_ w93]
              tunnel: w85 -> [_ w91]
              tunnel: [_ w90] -> w84
              frame False {
              }
              frame True {
                n155 = call "Enqueue.vi"("Message Data"=w93, "Message"="WriteEvtConfig", "MessageQueue"=w91) -> ("error out"=w90:errorcluster)  [unwired: 7 in, 1 out]
              }
            }
          }
          event User Event {
            n156 = event-data() -> ("ModuleID"=w98:i32, "Data"=w97:variant)  [unwired: 1 in]
            n157 = call <userlib>:"AddressedToThisModule.vi"("ModuleID"=w98, "ModuleAdmin"=w99) -> ("AddressedToThisInstance?"=w96:bool)  [unwired: 8 in, 1 out]
            n158 = case shown="True" w96 {
              tunnel: w97 -> [_ w103]
              tunnel: w95 -> [_ w102]
              tunnel: [_ w100] -> w94
              frame False {
              }
              frame True {
                n159 = call "Enqueue.vi"("Message Data"=w103, "Message"="ReadEvtConfig", "MessageQueue"=w102) -> ("error out"=w100:errorcluster)  [unwired: 7 in, 1 out]
              }
            }
          }
          event User Event {
            n160 = event-data() -> ("ModuleID"=w106:i32, "Data"=w105:variant)  [unwired: 1 in]
            n161 = call <userlib>:"AddressedToThisModule.vi"("ModuleID"=w106, "ModuleAdmin"=w107) -> ("AddressedToThisInstance?"=w109:bool)  [unwired: 8 in, 1 out]
            n162 = case shown="True" w109 {
              tunnel: [_ w112] -> w108
              tunnel: w105 -> [_ w111]
              tunnel: w104 -> [_ w110]
              frame False {
              }
              frame True {
                n163 = call "Enqueue.vi"("Message Data"=w111, "Message"="WriteTimeArray", "MessageQueue"=w110) -> ("error out"=w112:errorcluster)  [unwired: 7 in, 1 out]
              }
            }
          }
          event User Event {
            n164 = event-data() -> ("ModuleID"=w116:i32, "Data"=w115:variant)  [unwired: 1 in]
            n165 = call <userlib>:"AddressedToThisModule.vi"("ModuleID"=w116, "ModuleAdmin"=w118) -> ("AddressedToThisInstance?"=w119:bool)  [unwired: 8 in, 1 out]
            n166 = case shown="True" w119 {
              tunnel: [_ w122] -> w114
              tunnel: w117 -> [_ w121]
              tunnel: w115 -> [_ w120]
              frame False {
              }
              frame True {
                n167 = call "Enqueue.vi"("Message Data"=w120, "Message"="ReadTimeArray", "MessageQueue"=w121) -> ("error out"=w122:errorcluster)  [unwired: 7 in, 1 out]
              }
            }
          }
          event User Event {
            n168 = event-data() -> ("ModuleID"=w127:i32, "Data"=w128:variant)  [unwired: 1 in]
            n169 = call <userlib>:"AddressedToThisModule.vi"("ModuleID"=w127, "ModuleAdmin"=w126) -> ("AddressedToThisInstance?"=w129:bool)  [unwired: 8 in, 1 out]
            n170 = case shown="True" w129 {
              tunnel: [_ w132] -> w124
              tunnel: w128 -> [_ w131]
              tunnel: w125 -> [_ w130]
              frame False {
              }
              frame True {
                n171 = call "Enqueue.vi"("Message Data"=w131, "Message"="WriteEvtParams", "MessageQueue"=w130) -> ("error out"=w132:errorcluster)  [unwired: 7 in, 1 out]
              }
            }
          }
          event User Event {
            n172 = event-data() -> ("ModuleID"=w136:i32, "Data"=w138:variant)  [unwired: 1 in]
            n173 = call <userlib>:"AddressedToThisModule.vi"("ModuleID"=w136, "ModuleAdmin"=w137) -> ("AddressedToThisInstance?"=w139:bool)  [unwired: 8 in, 1 out]
            n174 = case shown="True" w139 {
              tunnel: [_ w142] -> w134
              tunnel: w138 -> [_ w141]
              tunnel: w135 -> [_ w140]
              frame False {
              }
              frame True {
                n175 = call "Enqueue.vi"("Message Data"=w141, "Message"="ReadEvtParams", "MessageQueue"=w140) -> ("error out"=w142:errorcluster)  [unwired: 7 in, 1 out]
              }
            }
          }
          event User Event {
            n176 = event-data() -> ("ModuleID"=w146:i32, "Data"=w148:variant)  [unwired: 1 in]
            n177 = call <userlib>:"AddressedToThisModule.vi"("ModuleID"=w146, "ModuleAdmin"=w147) -> ("AddressedToThisInstance?"=w149:bool)  [unwired: 8 in, 1 out]
            n178 = case shown="True" w149 {
              tunnel: [_ w152] -> w144
              tunnel: w148 -> [_ w151]
              tunnel: w145 -> [_ w150]
              frame False {
              }
              frame True {
                n179 = call "Enqueue.vi"("Message Data"=w151, "Message"="ReadWfrmParams", "MessageQueue"=w150) -> ("error out"=w152:errorcluster)  [unwired: 7 in, 1 out]
              }
            }
          }
          event User Event {
            n180 = event-data() -> ("ModuleID"=w156:i32, "Data"=w158:variant)  [unwired: 1 in]
            n181 = call <userlib>:"AddressedToThisModule.vi"("ModuleID"=w156, "ModuleAdmin"=w157) -> ("AddressedToThisInstance?"=w159:bool)  [unwired: 8 in, 1 out]
            n182 = case shown="True" w159 {
              tunnel: [_ w162] -> w154
              tunnel: w158 -> [_ w161]
              tunnel: w155 -> [_ w160]
              frame False {
              }
              frame True {
                n183 = call "Enqueue.vi"("Message Data"=w161, "Message"="WriteWfrmParams", "MessageQueue"=w160) -> ("error out"=w162:errorcluster)  [unwired: 7 in, 1 out]
              }
            }
          }
          event User Event {
            n184 = event-data() -> ("ModuleID"=w167:i32, "Data"=w165:variant)  [unwired: 1 in]
            n185 = call <userlib>:"AddressedToThisModule.vi"("ModuleID"=w167, "ModuleAdmin"=w168) -> ("AddressedToThisInstance?"=w169:bool)  [unwired: 8 in, 1 out]
            n186 = case shown="True" w169 {
              tunnel: [_ w172] -> w164
              tunnel: w166 -> [_ w171]
              tunnel: w165 -> [_ w170]
              frame False {
              }
              frame True {
                n187 = call "Enqueue.vi"("Message Data"=w170, "Message"="GetReportArray", "MessageQueue"=w171) -> ("error out"=w172:errorcluster)  [unwired: 7 in, 1 out]
              }
            }
          }
          event User Event {
            n188 = event-data() -> ("ModuleID"=w177:i32, "Data"=w175:variant)  [unwired: 1 in]
            n189 = call <userlib>:"AddressedToThisModule.vi"("ModuleID"=w177, "ModuleAdmin"=w178) -> ("AddressedToThisInstance?"=w179:bool)  [unwired: 8 in, 1 out]
            n190 = case shown="True" w179 {
              tunnel: [_ w182] -> w174
              tunnel: w176 -> [_ w181]
              tunnel: w175 -> [_ w180]
              frame False {
              }
              frame True {
                n191 = call "Enqueue.vi"("Message Data"=w180, "Message"="GetEvtSignal", "MessageQueue"=w181) -> ("error out"=w182:errorcluster)  [unwired: 7 in, 1 out]
              }
            }
          }
          event User Event {
            n192 = event-data() -> ("ModuleID"=w187:i32, "Data"=w185:variant)  [unwired: 1 in]
            n193 = call <userlib>:"AddressedToThisModule.vi"("ModuleID"=w187, "ModuleAdmin"=w188) -> ("AddressedToThisInstance?"=w189:bool)  [unwired: 8 in, 1 out]
            n194 = case shown="True" w189 {
              tunnel: [_ w192] -> w184
              tunnel: w186 -> [_ w191]
              tunnel: w185 -> [_ w190]
              frame False {
              }
              frame True {
                n195 = call "Enqueue.vi"("Message Data"=w190, "Message"="SendArbWfrm", "MessageQueue"=w191) -> ("error out"=w192:errorcluster)  [unwired: 7 in, 1 out]
              }
            }
          }
          event User Event {
            n196 = event-data() -> ("ModuleID"=w197:i32, "Data"=w195:variant)  [unwired: 1 in]
            n197 = call <userlib>:"AddressedToThisModule.vi"("ModuleID"=w197, "ModuleAdmin"=w198) -> ("AddressedToThisInstance?"=w199:bool)  [unwired: 8 in, 1 out]
            n198 = case shown="True" w199 {
              tunnel: [_ w202] -> w194
              tunnel: w196 -> [_ w201]
              tunnel: w195 -> [_ w200]
              frame False {
              }
              frame True {
                n199 = call "Enqueue.vi"("Message Data"=w200, "Message"="WriteStartEndTime", "MessageQueue"=w201) -> ("error out"=w202:errorcluster)  [unwired: 7 in, 1 out]
              }
            }
          }
          event User Event {
            n200 = event-data() -> ("ModuleID"=w207:i32, "Data"=w205:variant)  [unwired: 1 in]
            n201 = call <userlib>:"AddressedToThisModule.vi"("ModuleID"=w207, "ModuleAdmin"=w208) -> ("AddressedToThisInstance?"=w209:bool)  [unwired: 8 in, 1 out]
            n202 = case shown="True" w209 {
              tunnel: [_ w212] -> w204
              tunnel: w206 -> [_ w211]
              tunnel: w205 -> [_ w210]
              frame False {
              }
              frame True {
                n203 = call "Enqueue.vi"("Message Data"=w210, "Message"="ReadStartEndTime", "MessageQueue"=w211) -> ("error out"=w212:errorcluster)  [unwired: 7 in, 1 out]
              }
            }
          }
          event User Event {
            n204 = event-data() -> ("ModuleID"=w217:i32, "Data"=w215:variant)  [unwired: 1 in]
            n205 = call <userlib>:"AddressedToThisModule.vi"("ModuleID"=w217, "ModuleAdmin"=w218) -> ("AddressedToThisInstance?"=w219:bool)  [unwired: 8 in, 1 out]
            n206 = case shown="True" w219 {
              tunnel: [_ w222] -> w214
              tunnel: w216 -> [_ w221]
              tunnel: w215 -> [_ w220]
              frame False {
              }
              frame True {
                n207 = call "Enqueue.vi"("Message Data"=w220, "Message"="ConfigDlg", "MessageQueue"=w221) -> ("error out"=w222:errorcluster)  [unwired: 7 in, 1 out]
              }
            }
          }
          event User Event {
            n208 = event-data() -> ("ModuleID"=w228:i32, "Data"=w225:variant)  [unwired: 1 in]
            n209 = call <userlib>:"AddressedToThisModule.vi"("ModuleID"=w228, "ModuleAdmin"=w229) -> ("AddressedToThisInstance?"=w227:bool)  [unwired: 8 in, 1 out]
            n210 = case shown="True" w227 {
              tunnel: w226 -> [_ w233]
              tunnel: w225 -> [_ w232]
              tunnel: [_ w230] -> w224
              frame False {
              }
              frame True {
                n211 = call "Enqueue.vi"("Message Data"=w232, "Message"="ShowPanel", "MessageQueue"=w233) -> ("error out"=w230:errorcluster)  [unwired: 7 in, 1 out]
              }
            }
          }
          event Panel Close? {
            # "Hide on external launch"
            # "Discard the event so the QMH can complete"
            # "Called from another module or the QMH"
            n212 = event-data() -> ()  [unwired: 1 in, 1 out]
            n213 = property class="ModuleAdmin.lvclass"(reference=w240) -> ("Accessors:External Launch"=w235:bool)  [unwired: 1 in, 2 out]
            n214 = Bundle By Name(cluster=T3 {"Exit via Stop Module Req?"=FALSE, "Wait for Module to stop?"=FALSE, "ModuleAdmin"=refnum} ("Stop Argument"), "Wait for Module to stop?"=FALSE, "Exit via Stop Module Req?"=TRUE) -> (w241:T3)
            n215 = Select(t="HidePanel", s=w235, f="Exit" ("Message")) -> (s? t:f=w237:string)
            n216 = call "Enqueue.vi"("Message Data"=w241, "Message"=w237, "MessageQueue"=w246) -> ("error out"=w244:errorcluster)  [unwired: 7 in, 1 out]
            n217 = event-data("Discard?"=TRUE) -> ()  [unwired: 1 in, 1 out]
          }
        }
        n218 = call "ErrorHandler.vi"("error in (no error)"=w38, "MessageQueue"=w36) -> ("error out"=w37:errorcluster)  [unwired: 8 in, 1 out]
      }
    }
    frame Error {
      n219 = property class="ModuleAdmin.lvclass"(reference=w632) -> (reference out=w631:refnum<class "ModuleAdmin.lvclass">, "Accessors:CloneRegRef"=w629:refnum<data-value>, "Accessors:Module ID"=w628:i32)  [unwired: 1 in, 1 out]
      n220 = call <userlib>:"Remove.vi"("Module ID"=w628, "CloneRegRef"=w629) -> ("error out"=w634:errorcluster)  [unwired: 7 in, 2 out]
      n221 = flat-sequence {
        tunnel: w635 -> [w638]
        tunnel: w634 -> [_]
        tunnel: [w636] -> w633
        frame #0 {
          w637 = T13 2 items=["no dialog", "OK message", "continue or stop message", "OK message + warnings", "continue/stop + warnings"] ("type of dialog (OK msg:1)")
          n222 = call <vilib>:"Simple Error Handler.vi"("type of dialog (OK msg:1)"=w637, "error in (no error)"=w638) -> ("error out"=w636:errorcluster)  [unwired: 3 in, 4 out]
        }
      }
    }
  }
  n223 = Unregister For Events(event registration refnum=w4, error in=w5) -> (error out=w2:errorcluster)
  n224 = call "DestroyClone.vi"("error in (no error)"=w13, "Exit via Stop Module Req?"=w9, "Wait for Module to stop?"=w10, "ModuleAdmin"=w11) -> ("error out"=w12:errorcluster, "External Launch"=w8:bool)  [unwired: 5 in, 1 out]
  n225 = Release Queue(queue=w6, error in (no error)=w12) -> (error out=w7:errorcluster)  [unwired: 1 in, 2 out]
  n226 = Merge Errors(w2, w7) -> (w3:errorcluster)
  "error out" <- w3
  n227 = case shown="True" w8 {
    tunnel: w3 -> [_ w640]
    frame False {
    }
    frame True {
      n228 = control-ref of="This VI"() -> (w639:refnum<vi>)
      n229 = case shown="Error" w640 {
        tunnel: w639 -> [w641 w642]
        frame No Error {
          n230 = invoke class="VI" method="FP.Close"(reference=w641) -> ()  [unwired: 2 in, 3 out]
        }
        frame Error {
          n231 = invoke class="VI" method="FP.Open"(reference=w642, "Activate"=TRUE ("Activate?")) -> ()  [unwired: 3 in, 5 out]
        }
      }
    }
  }
